vi "defining input signal bandwidth.vi"() -> ()   [LabVIEW 2012]
uses:
  <vilib>/measure/maspectr.llb/FFT Power Spectrum and PSD for N Chan.vi
  <vilib>/measure/NI_MAPro.lvlib
panel:
  out "Waveform Graph 2":dynamicdata(graph)
  out "Waveform Graph":cluster{"f0":dbl, "df":dbl, "magnitude":dbl[]}[](graph)
  out "Power Spectrum / PSD":cluster{"f0":dbl, "df":dbl, "magnitude":dbl[]}[](array[cluster]) {"magnitude" format="%.2p"; "f0" format="%.2p"; "df" format="%.2p"}
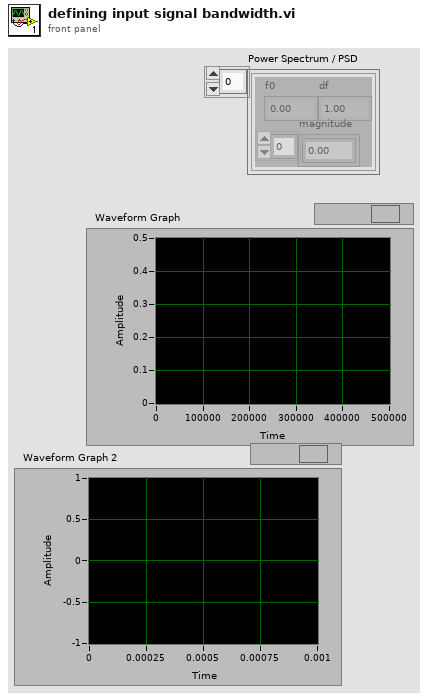
[diagram p1: front panel]
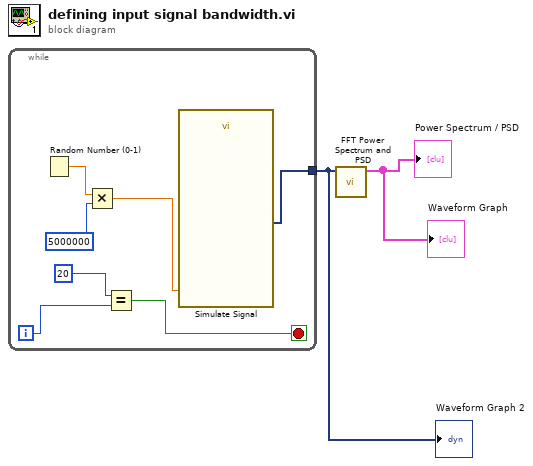
[diagram p0: block diagram]
diagram:
  n1 = while {
    tunnel: [w9] -> w1
    i -> [w4]
    stop <- w3 stop-if-true
    n2 = Random Number (0-1)() -> (number: 0 to 1=w8:dbl)
    n3 = Multiply(x=w8, y=5000000) -> (x*y=w6:dbl)
    n4 = Equal?(x=20, y=w4) -> (x = y?=w3:bool)
    n5 = call "Simulate Signal"("Frequency"=w6) -> ("Sine"=w9:dynamicdata)  [unwired: 13 in, 1 out]
  }
  "Waveform Graph 2" <- w1
  n6 = call-poly <vilib>:"FFT Power Spectrum and PSD.vi"("time signals"=w1) -> ("Power Spectrum / PSD"=→"Power Spectrum / PSD" →"Waveform Graph":cluster{"f0":dbl, "df":dbl, "magnitude":dbl[]}[])  [unwired: 7 in, 3 out]
